vi "3_5_1.vi"() -> ()   [LabVIEW 2012]
panel:
  out "Array 2":i32[](array[numeric])
  in  "element":dbl
  in  "Array":dbl[](array[numeric])
  in  "51-61":bool
  in  "stop":bool
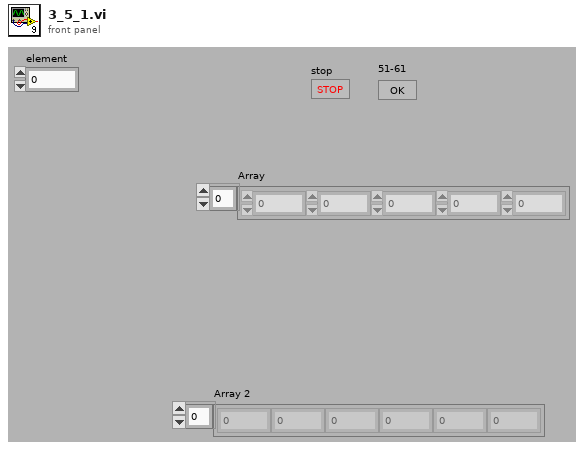
[diagram p1: front panel]
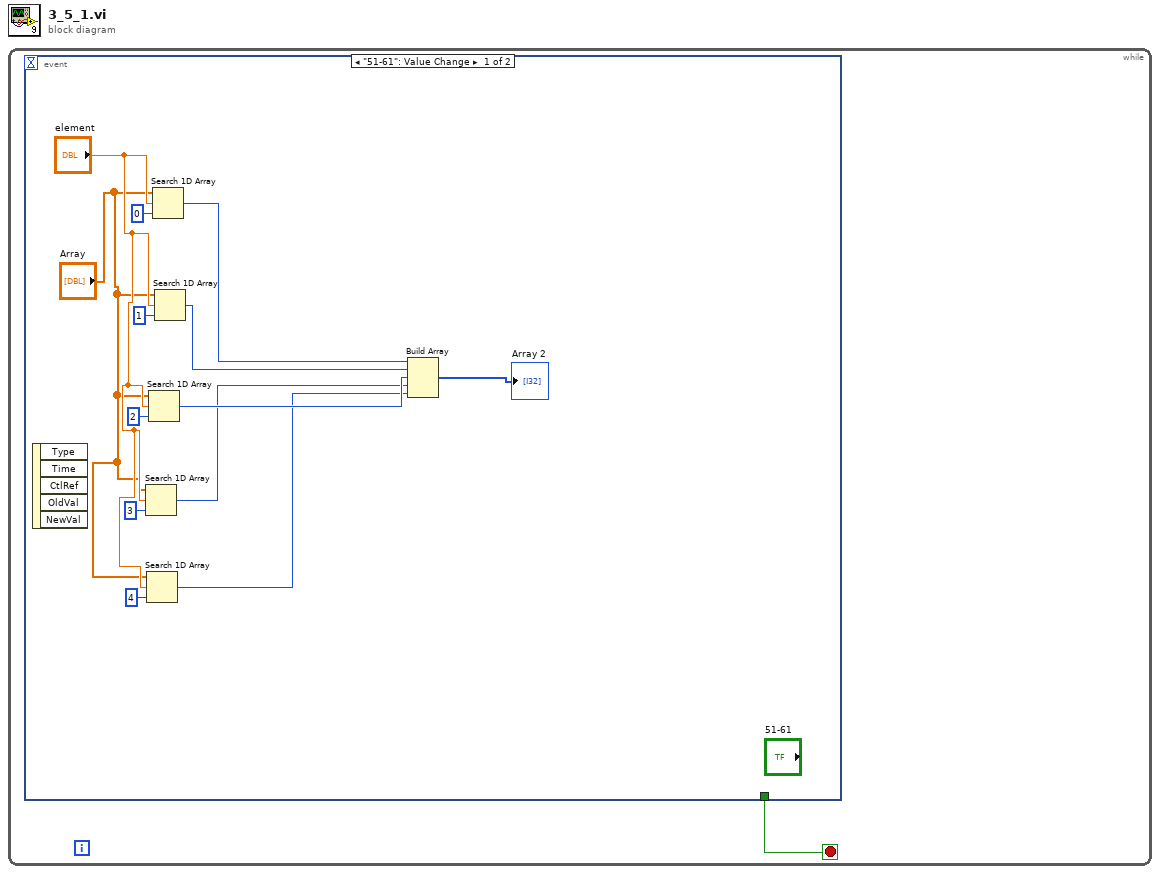
[diagram p0: block diagram]
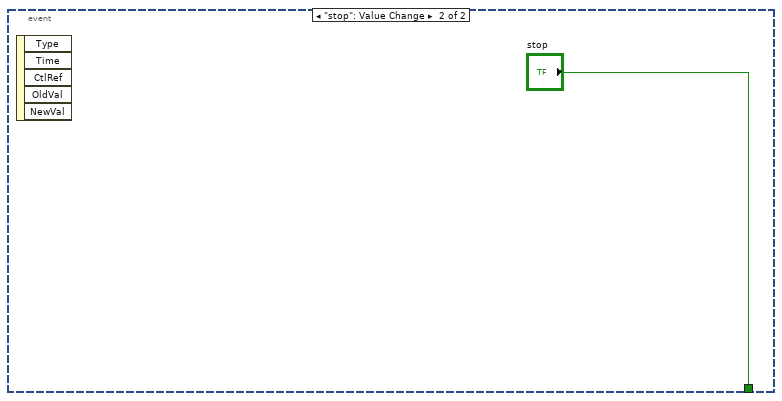
[diagram p2: hidden frame]
diagram:
  n1 = while {
    stop <- w1 stop-if-true
    n2 = event shown="[0] \"51-61\": Value Change" {
      selector: _ -> [_ _]
      dyn-events: _ -> [_ _]
      timeout: _ -> [_ _]
      tunnel: [_ "stop"] -> w1
      event "51-61": Value Change {
        n3 = event-data() -> ()  [unwired: 1 in, 5 out]
        n4 = Search 1D Array(1D array="Array", element="element", start index (0)=3) -> (index of element=w11:i32)
        n5 = Search 1D Array(1D array="Array", element="element", start index (0)=4) -> (index of element=w10:i32)
        n6 = Search 1D Array(1D array="Array", element="element", start index (0)=2) -> (index of element=w12:i32)
        n7 = Search 1D Array(1D array="Array", element="element", start index (0)=0) -> (index of element=w14:i32)
        n8 = Search 1D Array(1D array="Array", element="element", start index (0)=1) -> (index of element=w13:i32)
        n9 = Build Array(w14, w13, w12, w11, w10) -> (→"Array 2":i32[])
      }
      event "stop": Value Change {
        n10 = event-data() -> ()  [unwired: 1 in, 5 out]
      }
    }
  }
